vi "ACQ choose Chip Data_viewer.vi"(0 "Chip ID list":u32[](array[numeric]) format="%.0x", 5 "quants events per Chip":u32[](array[numeric]), 9 "summary IDs":string, 11 "Total of events":string) -> (4 "FullClose":bool, 8 "ChipID choosed":u16 format="%.0x")   [LabVIEW 2015, in "VIPM2.lvlib"]
doc: "Mostra en una nova finestra el resum d'events per Chip.\nRetorna el Chip escollit per al Data viewer."
uses:
  VIPM2.lvlib
panel:
  in  "Choose Array":T1(array[cluster])
  in  "Close button":bool
  # "Choose one Chip to watch its histograms"
  # "In green, events per Chip."
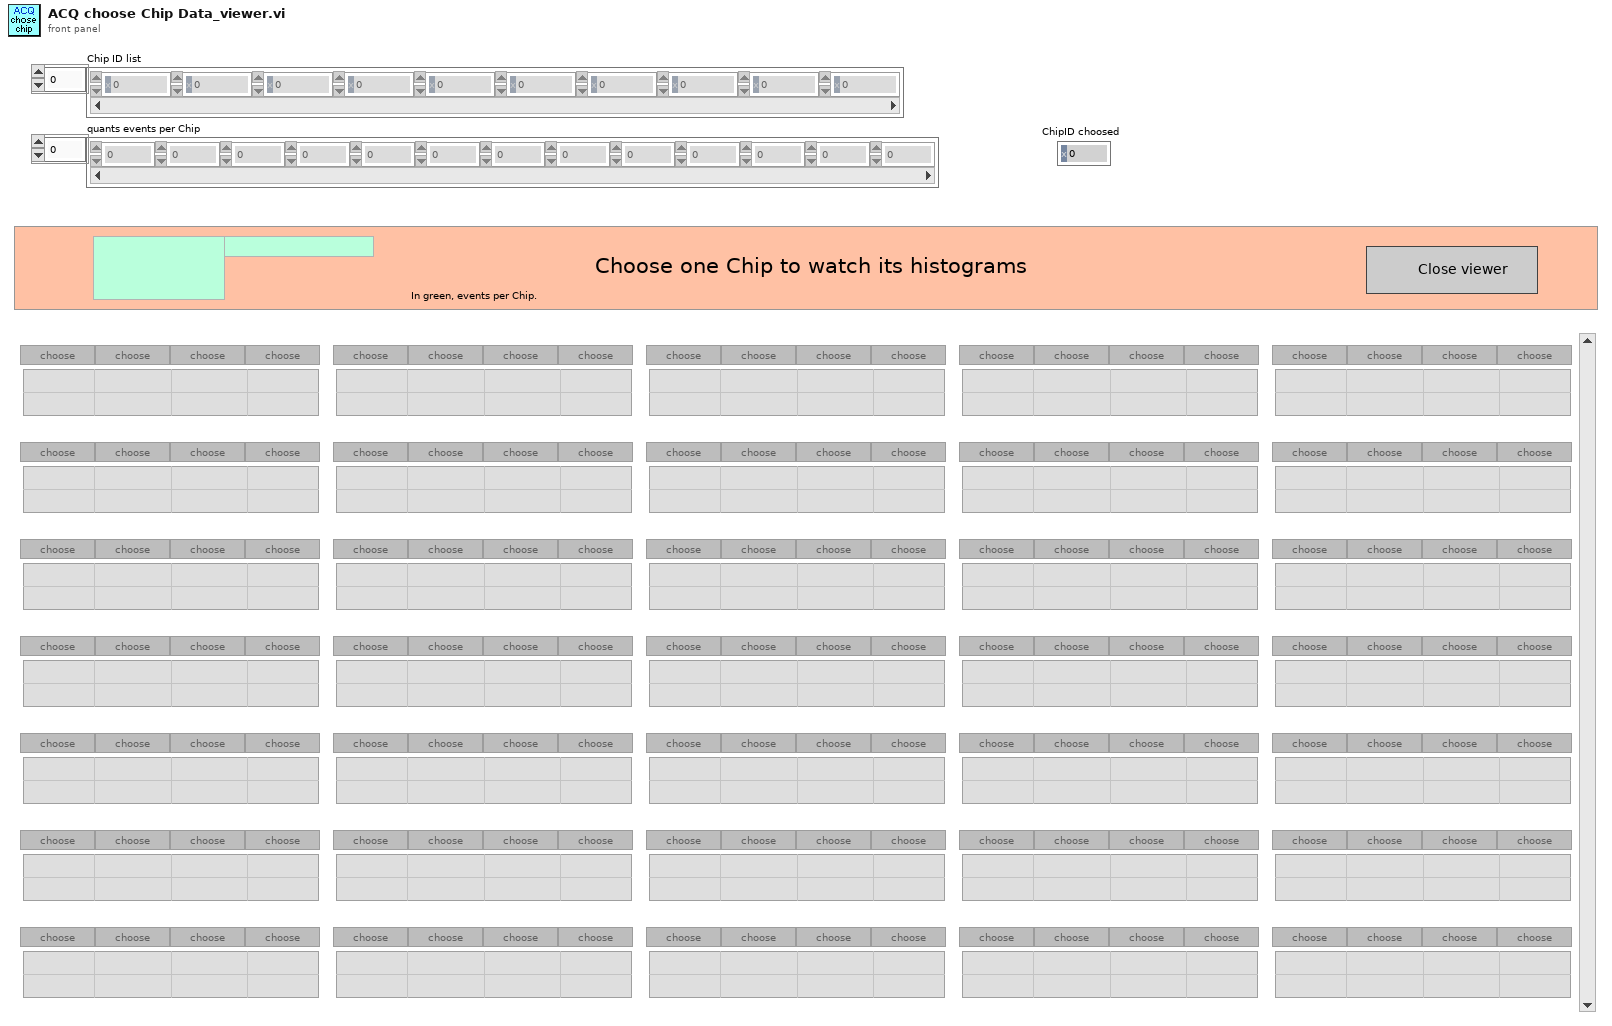
[diagram p1: front panel]
types:
  T1 = cluster{"SEL buttons":bool[], "Data table":string[][]}[][]
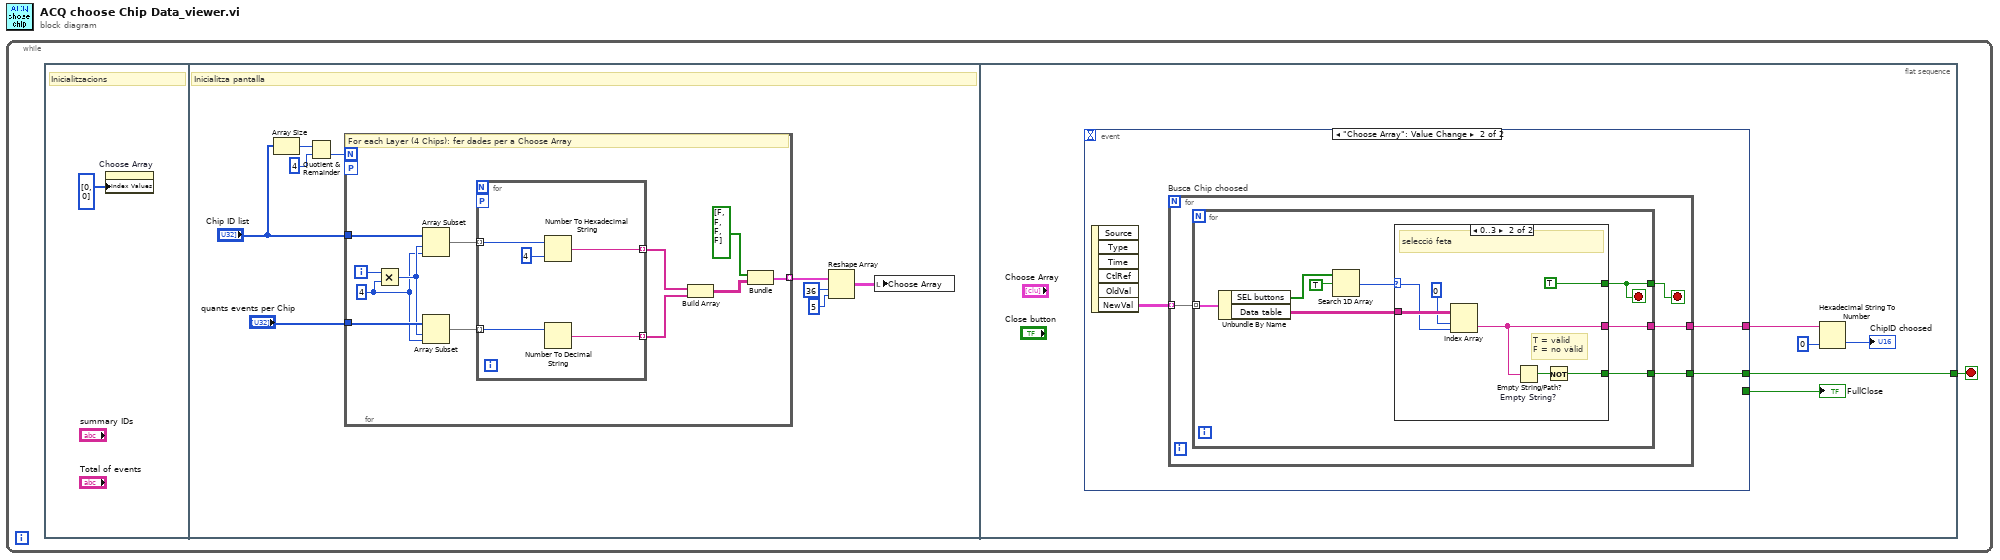
[diagram p0: block diagram]
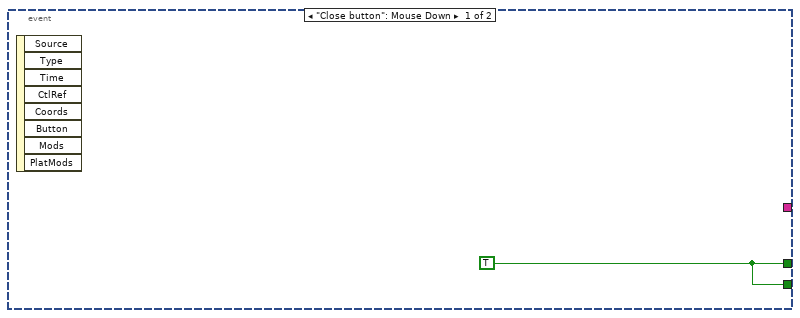
[diagram p2: hidden frame]
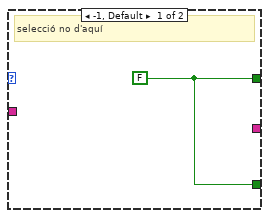
[diagram p3: hidden frame]
diagram:
  n1 = while {
    stop <- w1 stop-if-true
    n2 = flat-sequence {
      tunnel: [w33] -> w1
      frame #0 {
        # "Inicialitzacions"
        n3 = property on="Choose Array" class="Arr"("Index Values"=u32[] [0, 0]) -> ()  [unwired: 2 in, 2 out]
      }
      frame #1 {
        # "Inicialitza pantalla"
        n4 = Array Size(array="Chip ID list") -> (size(s)=w5:i32)
        n5 = Quotient & Remainder(x=w5, y=4) -> (floor(x/y)=w4:i32)  [unwired: 1 out]
        n6 = for {
          N: w4 -> [_]
          tunnel: "Chip ID list" -> [w23]
          tunnel: "quants events per Chip" -> [w22]
          tunnel: [w13] -> w8 mode=indexing
          workers-P: _ -> [_]
          i -> [w21]
          w19 = 4 ("y")
          # "For each Layer (4 Chips): fer dades per a Choose Array"
          n7 = Multiply(x=w21, y=w19) -> (x*y=w20:i32)
          n8 = Array Subset "Array Subset"(array=w23, index=w20, length=w19) -> (w18:u32[])
          n9 = Array Subset(array=w22, index=w20, length=w19) -> (w17:u32[])
          n10 = for {
            tunnel: w18 -> [w28] mode=indexing
            tunnel: w17 -> [w25] mode=indexing
            tunnel: [w26] -> w16 mode=indexing
            tunnel: [w24] -> w15 mode=indexing
            workers-P: _ -> [_]
            n11 = Number To Hexadecimal String(1:i16 4 ("width (-)"), 2:w28) -> (0:w26:string)
            n12 = Number To Decimal String(number=w25) -> (decimal integer string=w24:string)  [unwired: 1 in]
          }
          n13 = Build Array "Build Array"(w16, w15) -> (w14:string[][])
          n14 = Bundle("Choose Button"=bool[] [FALSE, FALSE, FALSE, FALSE], w14) -> (w13:cluster{"Choose Button":bool[], string[][]})  [unwired: 1 in]
        }
        n15 = Reshape Array "Reshape Array"(w8, 36 ("dimension size"), 5 ("dimension size")) -> (w7:cluster{"Choose Button":bool[], string[][]}[][])
        n16 = local write "Choose Array"(w7) -> ()
      }
      frame #2 {
        n17 = event shown="[1] \"Choose Array\": Value Change" {
          selector: _ -> [_ _]
          dyn-events: _ -> [_ _]
          timeout: _ -> [_ _]
          tunnel: [w34 w35] -> w33
          tunnel: [_ w36] -> w32
          tunnel: [w34 _] -> w29
          event "Close button": Mouse Down {
            w34 = TRUE
            n18 = event-data() -> ()  [unwired: 1 in, 8 out]
          }
          event "Choose Array": Value Change {
            n19 = event-data() -> ("NewVal"=w37:T1)  [unwired: 1 in, 5 out]
            n20 = for "Busca Chip choosed" {
              tunnel: w37 -> [w41] mode=indexing
              tunnel: [w39] -> w36
              tunnel: [w38] -> w35
              stop <- w40 stop-if-true
              n21 = for {
                tunnel: w41 -> [w49] mode=indexing
                tunnel: [w45] -> w40
                tunnel: [w43] -> w39
                tunnel: [w42] -> w38
                stop <- w45 stop-if-true
                n22 = Unbundle By Name(w49) -> ("SEL buttons"=w48:bool[], "Data table"=w44:string[][])
                n23 = Search 1D Array(1D array=w48, element=TRUE) -> (index of element=w46:i32)  [unwired: 1 in]
                n24 = case shown="0..3" w46 {
                  selector: w46 -> [_ w54]
                  tunnel: [w50 TRUE] -> w45
                  tunnel: w44 -> [_ w56]
                  tunnel: [_ w53] -> w43
                  tunnel: [w50 w51] -> w42
                  frame -1, Default {
                    w50 = FALSE
                    # "selecció no d'aquí"
                  }
                  frame 0..3 {
                    # "T = vàlid\nF = no vàlid"
                    # "selecció feta"
                    n25 = Index Array "Index Array"(array=w56, index (row)=0, index (col)=w54) -> (element=w53:string)
                    n26 = Empty String/Path? "Empty String?"(string/path=w53) -> (empty?=w52:bool)
                    n27 = Not(x=w52) -> (.not. x?=w51:bool)
                  }
                }
              }
            }
          }
        }
        "FullClose" <- w29
        n28 = Hexadecimal String To Number(string=w32, default (0uL)=u16 0 ("default (0 U32)")) -> (number=→"ChipID choosed":u16)  [unwired: 1 in, 1 out]
      }
    }
  }
